vi "Robot Global Data.vi"() -> ()   [LabVIEW 2013]
doc: "This global VI can contain as many global variables as you need. Place a control on the panel, give it a good name. To read or write to it from a VI, drag the icon to the diagram of that VI. You can also drag from the project. Click on the node to change which global you access. You shouldn't have multiple locations writing to a global or it will cause a race-condition."
uses:
  <vilib>/Rock Robotics/WPI/Camera/WPI_CameraImageSize.ctl
  <vilib>/Rock Robotics/WPI/DriverStation/WPI_DriverStationRobotMode2.ctl
panel:
  in  "Panic Mode":bool
  in  "Shoot Low?":bool
  in  "Conv OR 0":bool
  in  "Arm OR 0":bool=TRUE
  in  "Arm State":bool=TRUE
  in  "Reverse Shooter":bool
  in  "Conv Center":bool
  in  "Conv Axis":dbl
  in  "Arm Down S":bool
  in  "Arm OR":bool
  in  "Arm Motor OR":dbl
  in  "Reset Gyro":bool=TRUE
  in  "Shooter Mode":bool
  in  "Shoot?":bool
  in  "Center Cal'd":dbl
  in  "Gyro Yaw Rate":dbl
  in  "Gyro Angle":dbl
  in  "Disabled First Time":bool
  in  "Robot Mode":T1=enum."Teleop Disabled"
  in  "LED toggle rate (ms)":u32=100
  in  "image size":T2=enum."320x240"
  in  "Enable Vision":bool
  in  "Arm Down":bool
  in  "FC Angle":dbl
  in  "Auto FC":bool
  in  "Auton Gyro SP":dbl
  in  "Rotate By PID":dbl=-0.0
  in  "Reset Encoder PID":bool=TRUE
  in  "Rotate":dbl
  in  "Strafe":dbl
  in  "Fwd/Rev":dbl
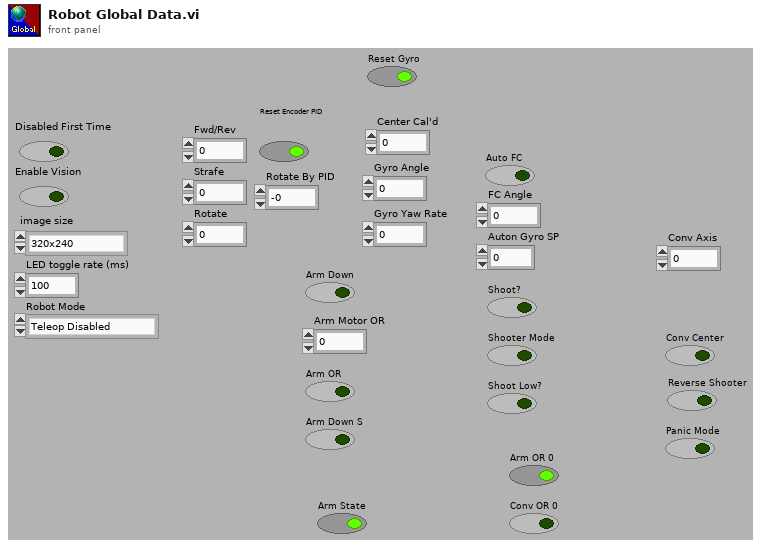
[diagram p1: front panel]
types:
  T1 = typedef "WPI_DriverStationRobotMode2.ctl" = enum16{"Autonomous Disabled", "Autonomous Enabled", "Teleop Disabled", "Teleop Enabled", "Timeout", "Finish", "Test Disabled", "Test Enabled"}
  T2 = typedef "WPI_CameraImageSize.ctl" = enum16{"640x480", "320x240", "160x120"}
diagram:
